vi "control_drona.vi"() -> ()   [LabVIEW 2015]
doc: "Very simple example showing how to use the base VIs to control the AR Drone and receive and display navigation data."
uses:
  <vilib>/LVH/AR Drone Toolkit/Decode NavData/Typedefs/NavData Demo.ctl
  <vilib>/LVH/AR Drone Toolkit/Type Defs/AR Drone Resource.ctl
  video_global.vi
  <vilib>/LVH/AR Drone Toolkit/AR Drone.lvlib
panel:
  out "Video Stream":picture
  out "AR Drone Resource":T1={"UDP Control Connection"=refnum, "UDP NavData Connection"=refnum, "UDP Video Connection (Drone 1.0)"=refnum, "TCP Video Connection (Drone 2.0)"=refnum, "TCP Control Port Connection"=refnum, "Drone IP address"="192.168.1.1", "Drone Command Port"=5556, "Drone NavData Port"=5554, "Drone Vid Stream Port"=5555, "Drone TCP Control Port"=5559, "Home IP address"="192.168.1.2", "Home Command Port"=56828, "Home NavData Port"=56829, "Home Vid Stream Port"=56830, "Drone Version"=0, "Drone Index"=0, "Command Sequence"=1}
  out "Numeric":i32
  out "x > y?":bool
  in  "stop 2":bool
  out "Battery Remaining":dbl(slide) scale=0.0..100.0
  out "NavData Out":T2
  in  "Control Cluster":T3 {"Yaw Speed" scale=-1.0..1.0; "Vertical Speed" scale=-1.0..1.0; "Pitch" scale=-1.0..1.0; "Roll" scale=-1.0..1.0}
  in  "stop":bool
  in  "Emergency Landing":bool
  in  "Take Off/Land":bool
  in  "Hover":bool
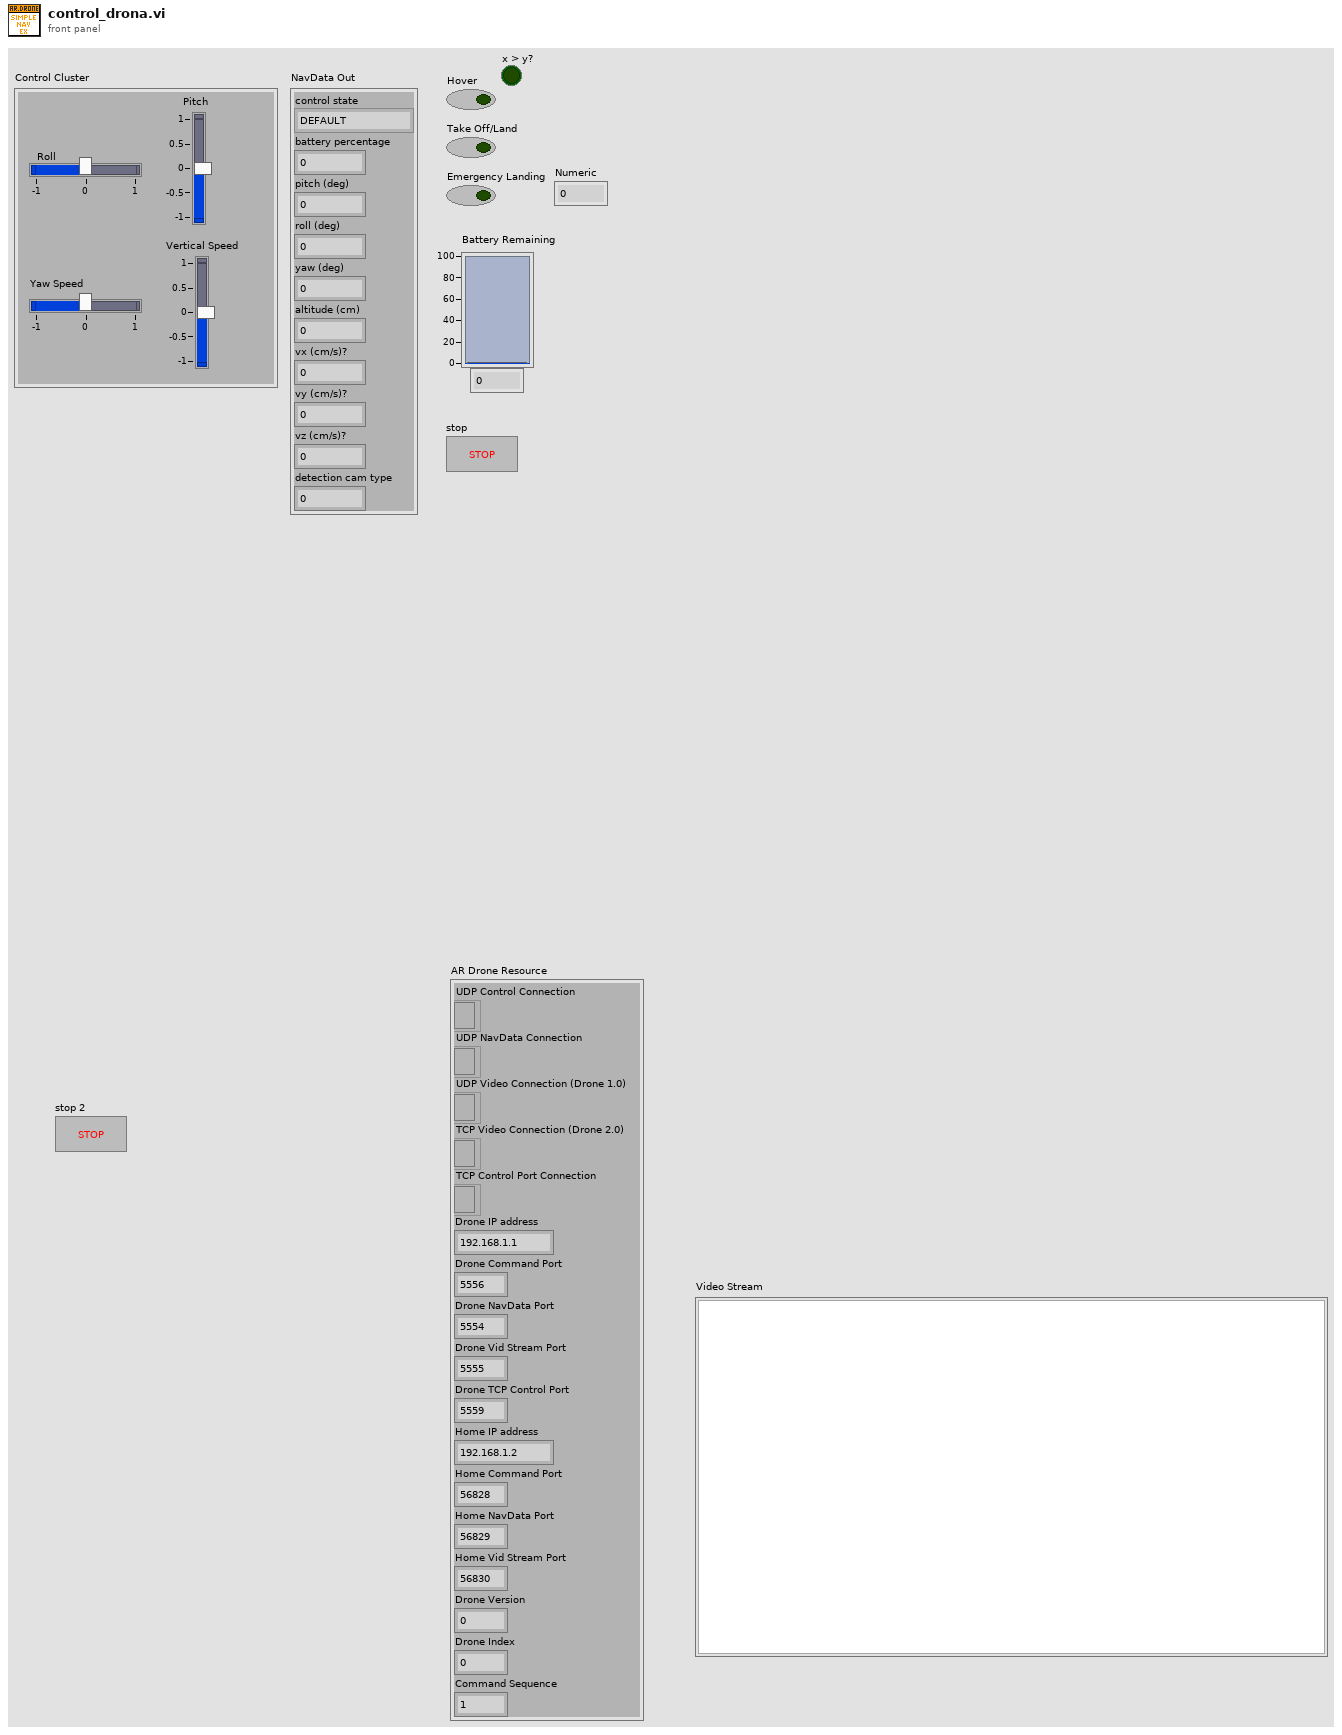
[diagram p1: front panel]
types:
  T1 = typedef "AR Drone.lvlib/AR Drone Resource.ctl" = cluster{"UDP Control Connection":refnum<k16>, "UDP NavData Connection":refnum<k16>, "UDP Video Connection (Drone 1.0)":refnum<k16>, "TCP Video Connection (Drone 2.0)":refnum<k5>, "TCP Control Port Connection":refnum<k5>, "Drone IP address":string, "Drone Command Port":u16, "Drone NavData Port":u16, "Drone Vid Stream Port":u16, "Drone TCP Control Port":u16, "Home IP address":string, "Home Command Port":u16, "Home NavData Port":u16, "Home Vid Stream Port":u16, "Drone Version":i32, "Drone Index":i32, "Command Sequence":i32}
  T2 = typedef "AR Drone.lvlib/NavData Demo.ctl" = cluster{"control state":enum32{"DEFAULT", "INIT", "LANDING", "FLYING", "HOVERING", "TEST", "TRANS_TAKEOFF", "TRANS_GOTOFIX", "TRANS_LANDING"}, "battery percentage":u32, "pitch (deg)":sgl, "roll (deg)":sgl, "yaw (deg)":sgl, "altitude (cm)":u32, "vx (cm/s)?":sgl, "vy (cm/s)?":sgl, "vz (cm/s)?":sgl, "detection cam type":u32}
  T3 = cluster{"Roll":sgl, "Pitch":sgl, "Vertical Speed":sgl, "Yaw Speed":sgl}
  T4 = cluster{"Drone IP address":string, "Home IP address":string, "Flight Mode":enum8{"OUTDOOR MODE", "INDOOR MODE"}, "Mounted Hull":enum8{"OUTDOOR HULL", "INDOOR HULL"}, "Video Camera":u8, "Max Altitude (m)":sgl, "Max Pitch and Roll Angle (deg)":sgl, "Max Vertical Speed (m/s)":sgl, "Max Yaw Speed (deg/s)":sgl}
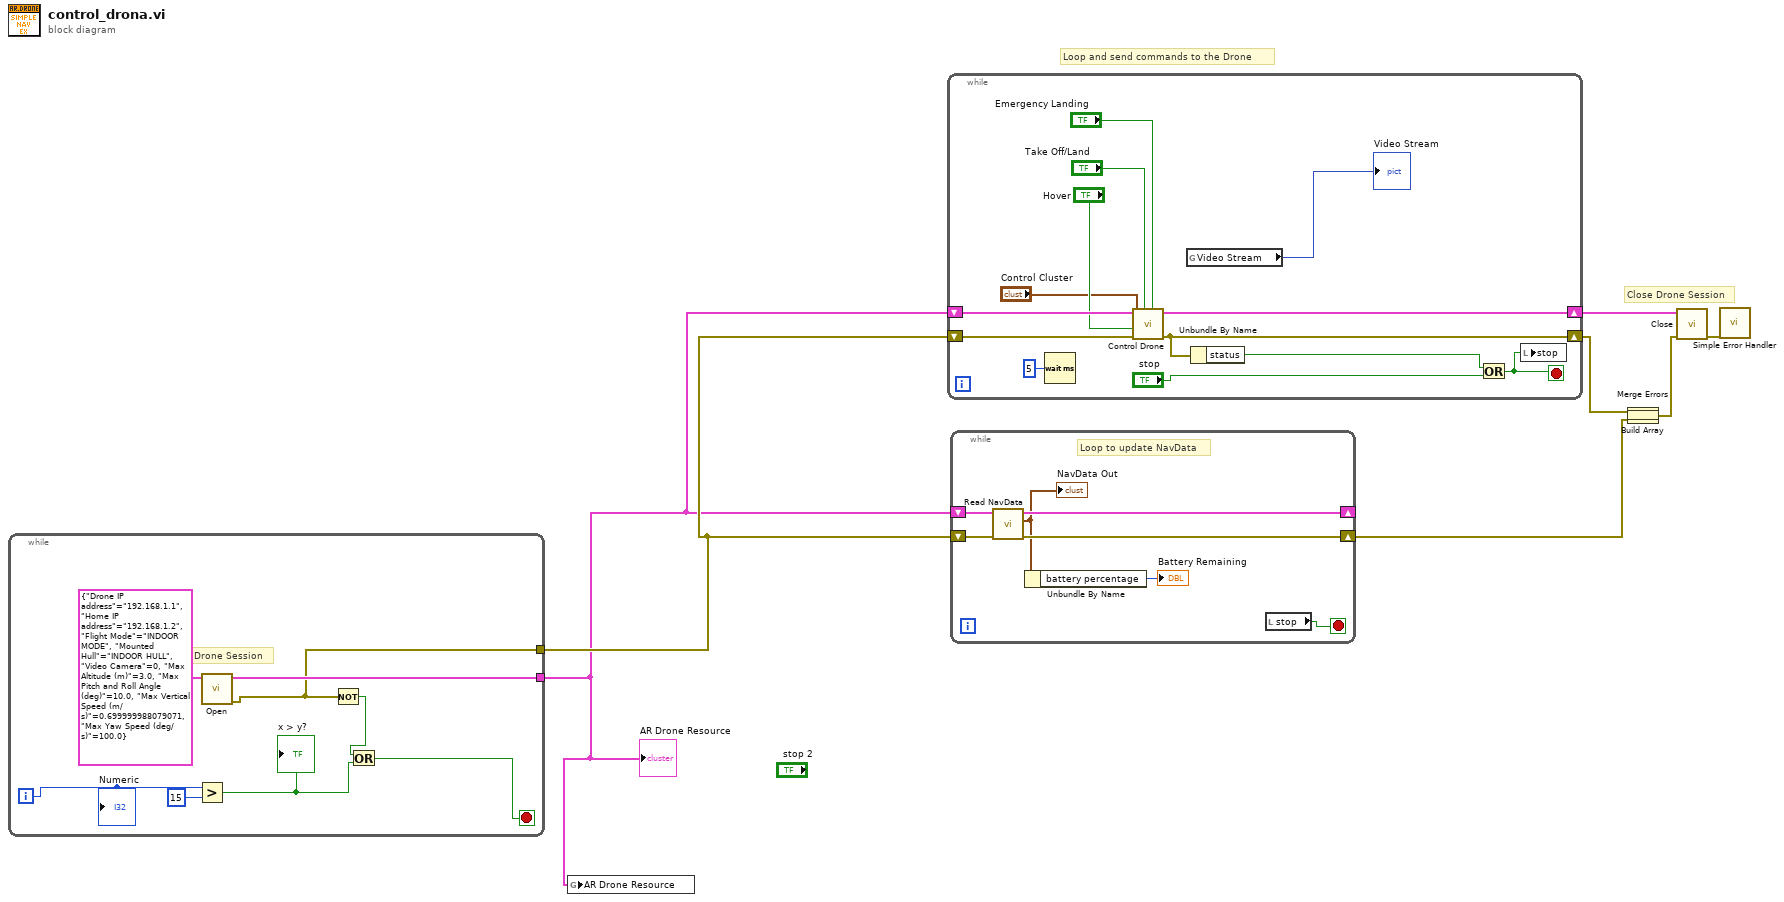
[diagram p0: block diagram]
diagram:
  # "Close Drone Session"
  # "Loop and send commands to the Drone"
  n1 = while {
    tunnel: [w10] -> w1
    tunnel: [w9] -> w2
    i -> [w15]
    stop <- w11 stop-if-true
    # "Open Drone Session"
    n2 = Greater?(x=w15, y=15) -> (0:w12:bool)
    "x > y?" <- w12
    n3 = call <vilib>:"Open.vi"("Setup Parameters"=T4 {"Drone IP address"="192.168.1.1", "Home IP address"="192.168.1.2", "Flight Mode"=enum."INDOOR MODE", "Mounted Hull"=enum."INDOOR HULL", "Video Camera"=0, "Max Altitude (m)"=3.0, "Max Pitch and Roll Angle (deg)"=10.0, "Max Vertical Speed (m/s)"=0.7, "Max Yaw Speed (deg/s)"=100.0}) -> ("error out"=w9:errorcluster, "AR Drone Resource"=w10:T1)  [unwired: 9 in]
    n4 = Not(x=w9) -> (.not. x?=w13:bool)
    n5 = Or(x=w13, y=w12) -> (x .or. y?=w11:bool)
    "Numeric" <- w15
  }
  "AR Drone Resource" <- w1
  n6 = global write "video_global.vi" "AR Drone Resource"(w1) -> ()
  n7 = while {
    shift-right: [w24] -> w8
    shift-left: w1 -> [w28]
    shift-right: [w19] -> w6
    shift-left: w2 -> [w29]
    stop <- w18 stop-if-true
    n8 = Wait (ms)(milliseconds to wait=u32 5) -> ()  [unwired: 1 out]
    n9 = call <vilib>:"Control Drone.vi"("Emergency Landing"="Emergency Landing", "Takeoff/Land"="Take Off/Land", "error in (no error)"=w29, "Hover"="Hover", "Control Cluster"="Control Cluster", "AR Drone Resource"=w28) -> ("error out"=w19:errorcluster, "AR Drone Resource Out"=w24:T1)  [unwired: 4 in]
    n10 = global read "video_global.vi" "Video Stream"() -> (→"Video Stream":picture)
    n11 = Unbundle By Name(w19) -> ("status"=w21:bool)
    n12 = Or(x=w21, y="stop") -> (x .or. y?=w18:bool)
    n13 = local write "stop"(w18) -> ()
  }
  n14 = while {
    shift-right: [w34] -> _
    shift-left: w1 -> [w35]
    shift-right: [w32] -> w7
    shift-left: w2 -> [w33]
    stop <- w36 stop-if-true
    # "Loop to update NavData"
    n15 = call <vilib>:"Read NavData.vi"("error in (no error)"=w33, "AR Drone Resource"=w35) -> ("error out"=w32:errorcluster, "NavData Out"=w31:T2, "AR Drone Resource Out"=w34:T1)  [unwired: 7 in]
    "NavData Out" <- w31
    n16 = Unbundle By Name(w31) -> ("battery percentage"=→"Battery Remaining":u32)
    n17 = local read "stop"() -> (w36:bool)
  }
  n18 = Build Array(w6, w7) -> (w3:errorcluster[])
  n19 = Merge Errors(w3) -> (w5:errorcluster)
  n20 = call <vilib>:"Close.vi"("error in (no error)"=w5, "AR Drone Resource"=w8) -> ("error out"=w4:errorcluster)  [unwired: 9 in]
  n21 = call <vilib>:"Simple Error Handler.vi"("error in (no error)"=w4) -> ()  [unwired: 4 in, 5 out]
